vi "Target Application (Main).vi"() -> ()   [LabVIEW 2013]
uses:
  SV B-M (Target) Class/SV B-M (Target).lvclass
panel:
  in  "Stop":bool
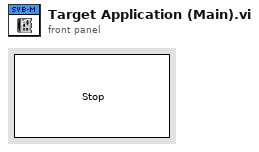
[diagram p1: front panel]
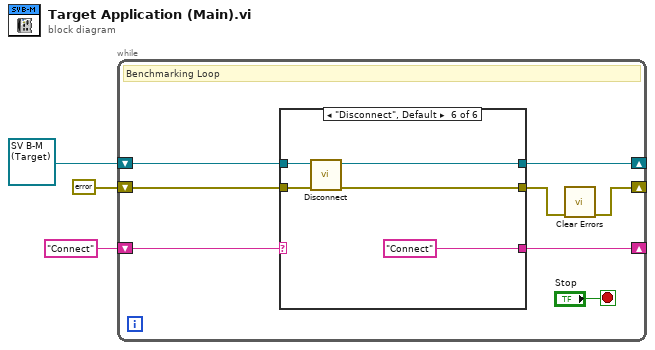
[diagram p0: block diagram]
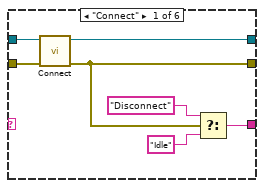
[diagram p2: hidden frame]
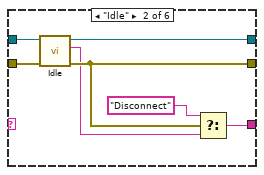
[diagram p3: hidden frame]
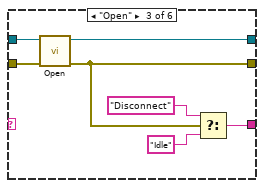
[diagram p4: hidden frame]
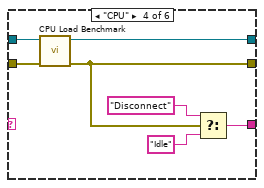
[diagram p5: hidden frame]
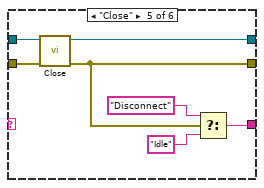
[diagram p6: hidden frame]
diagram:
  n1 = while {
    shift-right: [w6] -> _
    shift-left: "Connect" -> [w11]
    shift-right: [w4] -> _
    shift-left: errorcluster {"status"=FALSE, "code"=0, "source"=""} ("error constant") -> [w10]
    shift-right: [w9] -> _
    shift-left: refnum<class "SV B-M (Target).lvclass"> refnum ("SV B-M (Target).lvclass") -> [w8]
    stop <- "Stop" stop-if-true
    # "Benchmarking Loop"
    n2 = case shown="\"Disconnect\", Default" w11 {
      tunnel: w10 -> [w17 w24 w31 w38 w45 w50]
      tunnel: [w16 w23 w30 w37 w44 w49] -> w9
      tunnel: w8 -> [w18 w25 w32 w39 w46 w51]
      tunnel: [w13 w21 w27 w34 w41 w48] -> w5
      tunnel: [w12 w20 w26 w33 w40 "Connect"] -> w6
      frame "Connect" {
        n3 = call "Connect.vi"("error in (no error)"=w17, "SV B-M (Target) in"=w18) -> ("error out"=w13:errorcluster, "SV B-M (Target) out"=w16:refnum<class "SV B-M (Target).lvclass">)  [unwired: 8 in]
        n4 = Select(t="Disconnect", s=w13, f="Idle") -> (s? t:f=w12:string)
      }
      frame "Idle" {
        n5 = call "Idle.vi"("error in (no error)"=w24, "SV B-M (Target) in"=w25) -> ("error out"=w21:errorcluster, "Next State"=w19:string, "SV B-M (Target) out"=w23:refnum<class "SV B-M (Target).lvclass">)  [unwired: 7 in]
        n6 = Select(t="Disconnect", s=w21, f=w19) -> (s? t:f=w20:string)
      }
      frame "Open" {
        n7 = call "Open.vi"("error in (no error)"=w31, "SV B-M (Target) in"=w32) -> ("error out"=w27:errorcluster, "SV B-M (Target) out"=w30:refnum<class "SV B-M (Target).lvclass">)  [unwired: 8 in]
        n8 = Select(t="Disconnect", s=w27, f="Idle") -> (s? t:f=w26:string)
      }
      frame "CPU" {
        n9 = call "CPU Load Benchmark.vi"("error in (no error)"=w38, "SV B-M (Target) in"=w39) -> ("error out"=w34:errorcluster, "SV B-M (Target) out"=w37:refnum<class "SV B-M (Target).lvclass">)  [unwired: 8 in]
        n10 = Select(t="Disconnect", s=w34, f="Idle") -> (s? t:f=w33:string)
      }
      frame "Close" {
        n11 = call "Close.vi"("error in (no error)"=w45, "SV B-M (Target) in"=w46) -> ("error out"=w41:errorcluster, "SV B-M (Target) out"=w44:refnum<class "SV B-M (Target).lvclass">)  [unwired: 8 in]
        n12 = Select(t="Disconnect", s=w41, f="Idle") -> (s? t:f=w40:string)
      }
      frame "Disconnect", Default {
        n13 = call "Disconnect.vi"("error in (no error)"=w50, "SV B-M (Target) in"=w51) -> ("error out"=w48:errorcluster, "SV B-M (Target) out"=w49:refnum<class "SV B-M (Target).lvclass">)  [unwired: 8 in]
      }
    }
    n14 = call <vilib>:"Clear Errors.vi"("error in (no error)"=w5) -> ("error out"=w4:errorcluster)  [unwired: 6 in]
  }
